vi "Tenary Operator.vi"() -> ()   [LabVIEW 2020]
panel:
  out "String":string
  in  "Boolean":bool
  # "Tenary Operator"
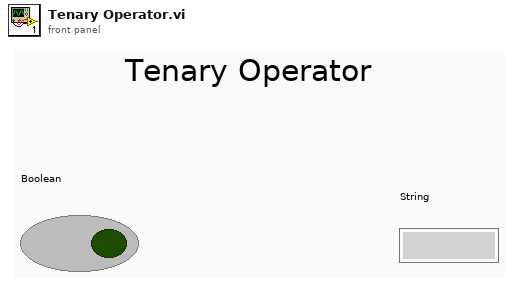
[diagram p1: front panel]
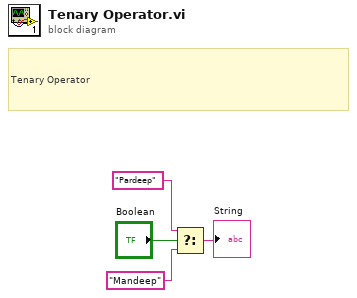
[diagram p0: block diagram]
diagram:
  # "Tenary Operator"
  n1 = Select(t="Pardeep", s="Boolean", f="Mandeep") -> (s? t:f=→"String":string)
